vi "Init Data.vi"(8 "error in (no error)":errorcluster, 11 "Device Reference in":T5 format="%.0x") -> (0 "error out":errorcluster, 2 "Compiled.Settings":T1 {"Tx Packet Info"."Endianness" items=["big-endian"=0, "little-indian"=2]; "Rx Packet Info"."Endianness" items=["big-endian"=0, "little-indian"=2]}, 3 "Device Reference out":T5 format="%.0x")   [LabVIEW 2016, in "UDP-Custom-Device Engine.lvlib"]
uses:
  UDP-Custom-Device Engine.lvlib
  <vilib>/NI Veristand/Custom Device API/Custom Device Item Ref.ctl
  Shared/Compiled.Settings.ctl
  Shared/Rx.PacketInfo.ctl
  System Explorer/Types/Channel Data Type.ctl
  Shared/Tx.PacketInfo.ctl
  Shared/Constants.vi
  <vilib>/NI Veristand/Custom Device API/Get Item Property (Variant).vi
  <vilib>/NI VeriStand/Custom Device API/Custom Device API.lvlib
  Shared/UDP-Custom-Device Shared.lvlib
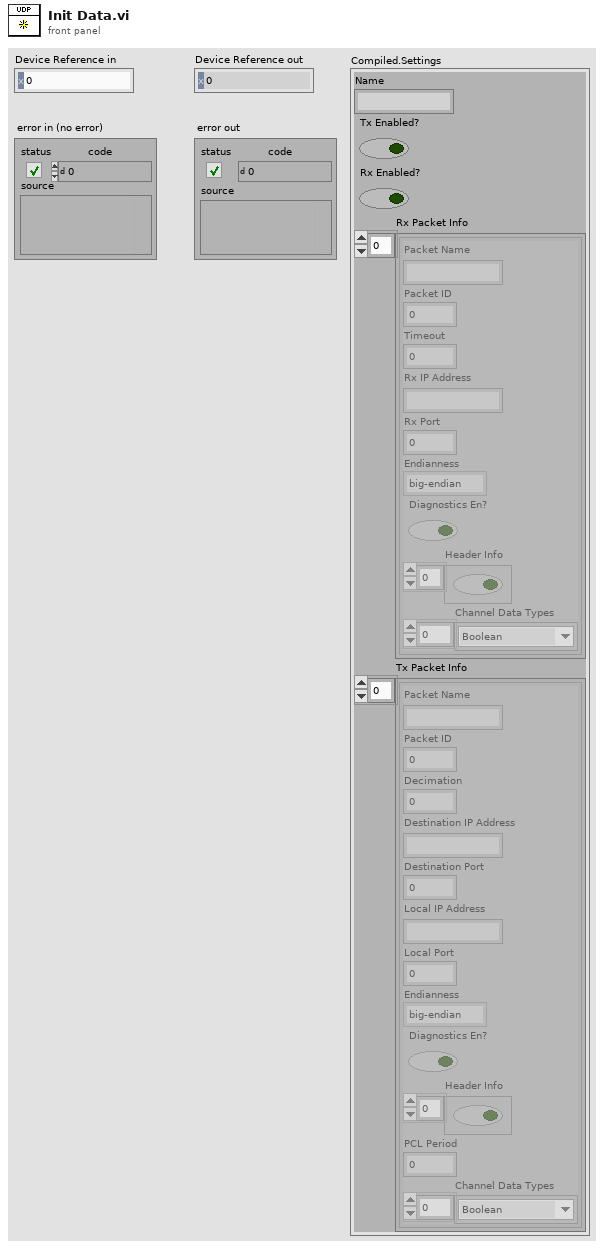
[diagram p1: front panel]
types:
  T1 = typedef "UDP-Custom-Device Shared.lvlib/Compiled.Settings.ctl" = cluster{"Name":string, "Tx Enabled?":bool, "Rx Enabled?":bool, "Rx Packet Info":T2[], "Tx Packet Info":T4[]}
  T2 = typedef "UDP-Custom-Device Shared.lvlib/Rx.PacketInfo.ctl" = cluster{"Packet Name":string, "Packet ID":i32, "Timeout":i32, "Rx IP Address":string, "Rx Port":i32, "Endianness":u16, "Diagnostics En?":bool, "Header Info":bool[], "Channel Data Types":T3[]}
  T3 = typedef "UDP-Custom-Device Shared.lvlib/Channel Data Type.ctl" = enum16{"Boolean", "Single"}
  T4 = typedef "UDP-Custom-Device Shared.lvlib/Tx.PacketInfo.ctl" = cluster{"Packet Name":string, "Packet ID":i32, "Decimation":i32, "Destination IP Address":string, "Destination Port":i32, "Local IP Address":string, "Local Port":i32, "Endianness":u16, "Diagnostics En?":bool, "Header Info":bool[], "PCL Period":u32, "Channel Data Types":T3[]}
  T5 = typedef "Custom Device API.lvlib/Custom Device Item Ref.ctl" = u64
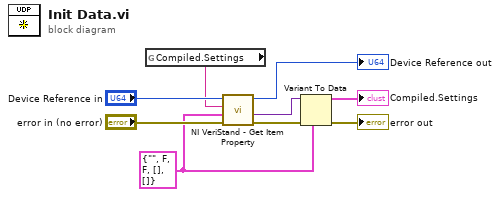
[diagram p0: block diagram]
diagram:
  w4 = T1 {"Name"="", "Tx Enabled?"=FALSE, "Rx Enabled?"=FALSE, "Rx Packet Info"=[], "Tx Packet Info"=[]} ("Compiled.Settings")
  n1 = global read "Constants.vi" "Compiled.Settings"() -> (w7:string)
  n2 = call-poly <vilib>:"NI VeriStand - Get Item Property.vi"("error in (no error)"="error in (no error)", "Default Value"=w4, "Property Name"=w7, "Item Ref in"="Device Reference in") -> ("error out"=w6:errorcluster, "Value"=w5:variant, "Item Ref out"=→"Device Reference out":T5)  [unwired: 4 in, 1 out]
  n3 = Variant To Data(error in=w6, type=w4, Variant=w5) -> (data=→"Compiled.Settings":T1, error out=→"error out":errorcluster)
